vi "Write Display.vi"(8 "error in (no error)":errorcluster, 9 "Display On":bool, 10 "VISA resource name in":refnum<visa-resource-name>, 11 "LCD-I2C in":refnum<class "LCD-I2C.lvclass">) -> (0 "error out":errorcluster, 2 "VISA resource name":refnum<visa-resource-name>, 3 "LCD-I2C out":refnum<class "LCD-I2C.lvclass">)   [LabVIEW 2023, in "CTI-Visa-DeviceLib.lvlib" / "LCD-I2C.lvclass"]
uses:
  LCD-I2C.lvclass
  LCD-I2C.lvclass/LCD-I2C.ctl
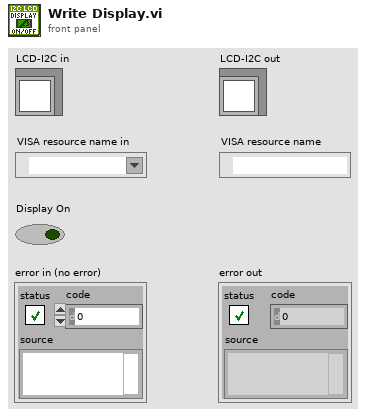
[diagram p1: front panel]
types:
  T1 = typedef "CTI-Visa-DeviceLib.lvlib/LCD-I2C.lvclass/Display Control.ctl" = cluster{"Blink On":bool, "Cursor On":bool, "Display On":bool}
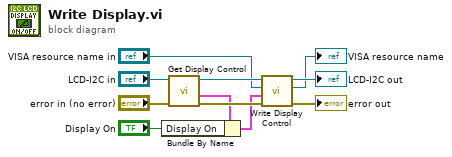
[diagram p0: block diagram]
diagram:
  n1 = call "Get Display Control.vi"("error in (no error)"="error in (no error)", "LCD-I2C in"="LCD-I2C in") -> ("error out"=w11:errorcluster, "Display Control"=w7:T1, "LCD-I2C out"=w9:refnum<class "LCD-I2C.lvclass">)  [unwired: 7 in]
  n2 = Bundle By Name(cluster=w7, "Display On"="Display On") -> (w4:T1)
  n3 = call "Write Display Control.vi"("error in (no error)"=w11, "Display Control"=w4, "VISA resource name in"="VISA resource name in", "LCD-I2C in"=w9) -> ("error out"=→"error out":errorcluster, "VISA resource name"=→"VISA resource name":refnum<visa-resource-name>, "LCD-I2C out"=→"LCD-I2C out":refnum<class "LCD-I2C.lvclass">)  [unwired: 5 in]
